vi "Pointer.In-Place Read (U8).vi"(8 "error in (no error)":errorcluster, 10 "value in":u8, 11 "pointer in":u64) -> (0 "error out":errorcluster, 2 "value out":u8, 3 "pointer out":u64)   [LabVIEW 2016, in "VeriStand Data.lvlib"]
doc: "Reads a value, in-place, from the provided <B>pointer</B>."
uses:
  VeriStand Data.lvlib
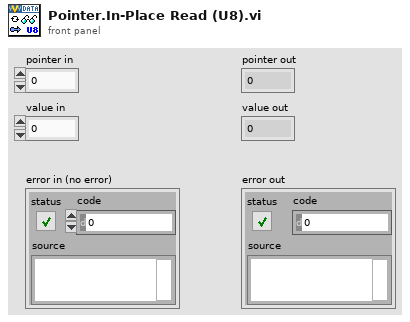
[diagram p1: front panel]
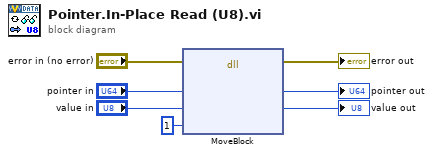
[diagram p0: block diagram]
diagram:
  n1 = dll-call lib="LabVIEW" fn="MoveBlock"(error in="error in (no error)", "ps"="pointer in", "pd"="value in", "size"=u64 1) -> (error out=→"error out":errorcluster, "ps"=→"pointer out":u64, "pd"=→"value out":u8)  [unwired: 4 in, 1 out]
